vi "MGI Set Custom Error Codes.vi"(9 "Custom Name[i] (Default Set)":string[](array[string]), 10 "Custom Code[i] (Default Set)":i32[](array[numeric])=[0], 11 "MGI Error Reporter Base In":refnum<class "MGI Error Reporter Base.lvclass">) -> (3 "MGI Error Reporter Base Out":refnum<class "MGI Error Reporter Base.lvclass">)   [LabVIEW 2016, in "MGI Error Reporter Base.lvclass"]
doc: "Set the custom error codes that will be used by the Error Reporter. The Custom Name array should contain short single line descriptions of each code.\n\nAuthored by Shawn Walpole\nsupport@mooregoodideas.com\nwww.mooregoodideas.com\n\nCopyright (c) 2013, Moore Good Ideas, Inc.\n\nAll rights reserved.\n\nRedistribution and use in source and binary forms, with or without modification, are permitted provided that the following conditions are met:\n\n * Redistributions of source code must retain the above copyright notice, this list of conditions and the following disclaimer.\n * Redistributions in binary form must reproduce the above copyright notice, this list of conditions and the following disclaimer in the documentation and/or other materials provided with the distribution.\n * Neither the name of Moore Good Ideas, Inc. nor the names of its contributors may be used to endorse or promote products derived from this software without specific prior written permission.\n\nTHIS SOFTWARE IS PROVIDED BY THE COPYRIGHT HOLDERS AND CONTRIBUTORS \"AS IS\" AND ANY EXPRESS OR IMPLIED WARRANTIES, INCLUDING, BUT NOT LIMITED TO, THE IMPLIED WARRANTIES OF MERCHANTABILITY AND FITNESS FOR A PARTICULAR PURPOSE ARE DISCLAIMED. IN NO EVENT SHALL THE COPYRIGHT OWNER OR CONTRIBUTORS BE LIABLE FOR ANY DIRECT, INDIRECT, INCIDENTAL, SPECIAL, EXEMPLARY, OR CONSEQUENTIAL DAMAGES (INCLUDING, BUT NOT LIMITED TO, PROCUREMENT OF SUBSTITUTE GOODS OR SERVICES; LOSS OF USE, DATA, OR PROFITS; OR BUSINESS INTERRUPTION) HOWEVER CAUSED AND ON ANY THEORY OF LIABILITY, WHETHER IN CONTRACT, STRICT LIABILITY, OR TORT (INCLUDING NEGLIGENCE OR OTHERWISE) ARISING IN ANY WAY OUT OF THE USE OF THIS SOFTWARE, EVEN IF ADVISED OF THE POSSIBILITY OF SUCH DAMAGE."
uses:
  <userlib>/_MGI/Error Reporter/MGI Error Reporter Base/MGI Error Reporter Base.lvclass
  <userlib>/_MGI/Error Reporter/MGI Error Reporter Base/MGI Error Reporter Base.lvclass/MGI Error Reporter Base.ctl
  <vilib>/Utility/VariantDataType/VariantType.lvlib
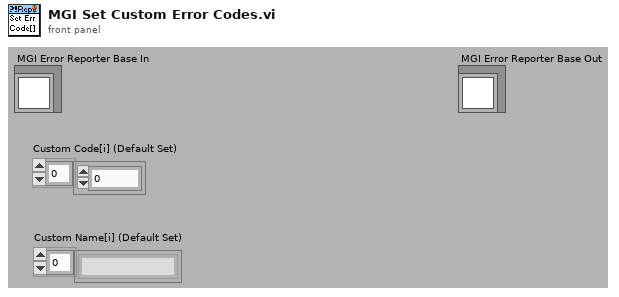
[diagram p1: front panel]
types:
  T1 = enum16{"No error", "Argument error", "Memory is full", "Out of zone", "End of file", "File already open", "Generic file I/O error", "File not found", "File permission error", "Disk is full", "Duplicate path", "Too many files open", "System feature not enabled", "Resource file not found", "Cannot add resource", "Resource not found", "Image not found", "Image memory error", "Pen does not exist", "Config type invalid", "Config token not found", "Config parse error", "Config memory error", "Bad external code format", "Bad external code offset", "External code not present", "Null window", "Destroy window error", "Null menu", "Print aborted", "Bad print record", "Print driver error", "Windows error during printing", "Memory error during printing", "Print dialog error", "Generic print error", "Invalid device refnum", "Device not found", "Device parameter error", "Device unit error", "Cannot open device", "Device call aborted", "Generic error", "Cancelled by user", "Object ID too low", "Object ID too high", "Object not in heap", "Unknown heap", "Unknown object (invalid DefProc)", "Unknown object (DefProc not in table)", "Message out of range", "Invalid (null) method", "Unknown message", "Manager call not supported", "Bad address", "Network operation in progress", "Network operation timed out", "Connection is busy", "Network attribute not supported", "Network error", "Address in use", "System out of memory", "Connection aborted", "Connection refused", "Not connected", "Already connected", "Connection closed", "Initialization error (interapplication manager)", "Bad occurrence", "Wait on unbound occurrence handler", "Occurrence queue overflow", "Datalog type conflict", "Unused", "Unrecognized type (interapplication manager)", "Memory corrupt", "Failed to make temporary DLL", "Old CIN version", "Drag socket not found", "Failed to load drop-object", "Failed to register OLE object", "Failed to release OLE object", "Format specifier type mismatch", "Unknown format specifier", "Too few format specifiers", "Too many format specifiers", "Scan failed", "Newer CIN version", "OLE Convert", "Runtime menu error", "Password tampered", "Unknown error code"}
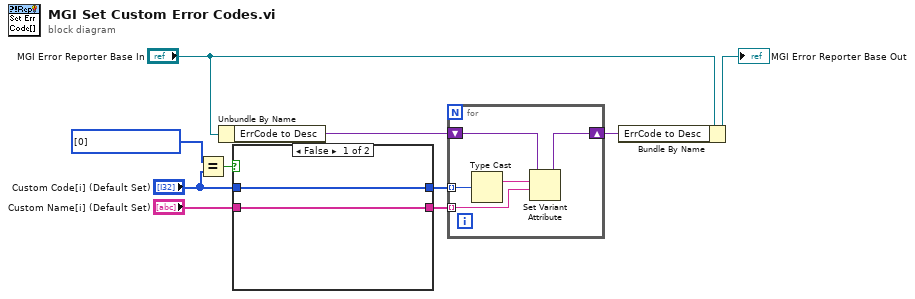
[diagram p0: block diagram]
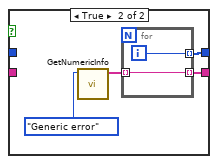
[diagram p2: hidden frame]
diagram:
  n1 = Equal?(x=i32[] [0] ("Custom Code[i] (Don't change)"), y="Custom Code[i] (Default Set)") -> (x = y?=w1:bool)
  n2 = Unbundle By Name("MGI Error Reporter Base In") -> ("ErrCode to Desc"=w9:variant)
  n3 = case shown="False" w1 {
    tunnel: "Custom Code[i] (Default Set)" -> [w12 _]
    tunnel: [w12 w13] -> w4
    tunnel: "Custom Name[i] (Default Set)" -> [w11 _]
    tunnel: [w11 w14] -> w2
    frame False {
    }
    frame True {
      n4 = call <vilib>:"GetNumericInfo.vi"("Variant"=T1."Generic error" ("Reserved Error Code (Generic error)")) -> ("EnumNames"=w15:string[])  [unwired: 1 in, 9 out]
      n5 = for {
        tunnel: [w18] -> w13 mode=indexing
        tunnel: w15 -> [w17] mode=indexing
        tunnel: [w17] -> w14 mode=indexing
        i -> [w18]
      }
    }
  }
  n6 = for {
    shift-right: [w22] -> w6
    shift-left: w9 -> [w23]
    tunnel: w2 -> [w21] mode=indexing
    tunnel: w4 -> [w20] mode=indexing
    n7 = Type Cast(x=w20) -> (*(type *) &x=w19:string)  [unwired: 1 out]
    n8 = Set Variant Attribute(Variant=w23, name=w19, value=w21) -> (Variant out=w22:variant)  [unwired: 1 in, 2 out]
  }
  n9 = Bundle By Name(cluster="MGI Error Reporter Base In", "ErrCode to Desc"=w6) -> (→"MGI Error Reporter Base Out":refnum<class "MGI Error Reporter Base.lvclass">)
